vi "Open Relays.vi"(8 "error in (no error)":errorcluster, 9 "nodePath":string, 10 "NIVS.System Definition Root":refnum<k24>, 11 "WorkspaceManager in":T1) -> (0 "error out":errorcluster, 3 "WorkspaceManager out":T1)   [LabVIEW 2013]
uses:
  NationalInstruments.VeriStand.SystemStorage
  <vilib>/NI Veristand/Execution/Workspace/WorkspaceAPI.ctl
  NationalInstruments.VeriStand.ClientAPI
  NationalInstruments.VeriStand
  <vilib>/NI Veristand/Execution/Workspace/NI VeriStand - Set Single Channel Value.vi
  <vilib>/NI Veristand/Execution/Workspace/NI_VS Workspace ExecutionAPI.lvlib
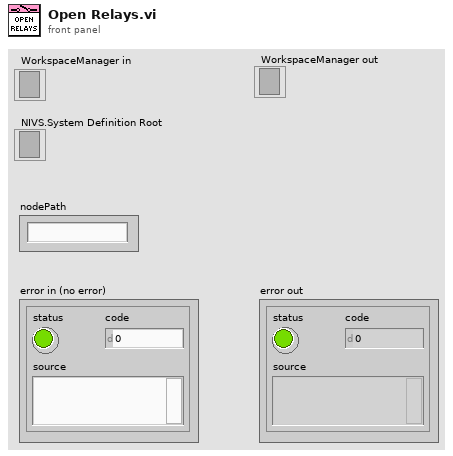
[diagram p1: front panel]
types:
  T1 = typedef "NI_VS Workspace ExecutionAPI.lvlib/WorkspaceAPI.ctl" = refnum<k24>
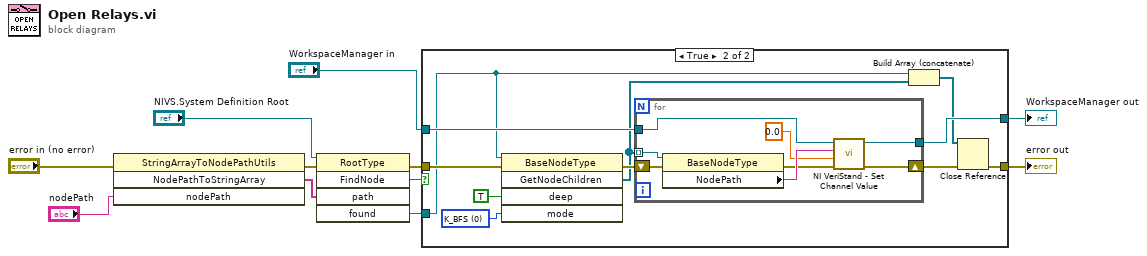
[diagram p0: block diagram]
diagram:
  n1 = invoke class="StringArrayToNodePathUtils" method="NodePathToStringArray"(error in="error in (no error)", "nodePath"="nodePath") -> (error out=w10:errorcluster, "NodePathToStringArray"=w11:string[])  [unwired: 2 in, 2 out]
  n2 = invoke class="RootType" method="FindNode"(reference="NIVS.System Definition Root", error in=w10, "path"=w11) -> (error out=w9:errorcluster, "FindNode"=w6:bool, "found"=w5:refnum<k24>)  [unwired: 2 in, 2 out]
  n3 = case shown="True" w6 {
    tunnel: w9 -> [w13 w24]
    tunnel: w5 -> [_ w16]
    tunnel: "WorkspaceManager in" -> [w12 w20]
    tunnel: [w12 w19] -> w3
    tunnel: [w13 w17] -> w2
    frame False {
    }
    frame True {
      w22 = 0 items=["K_BFS", "K_DFS", "K_CHILDONLY", "K_UP"] ("mode")
      n4 = invoke class="BaseNodeType" method="GetNodeChildren"(reference=w16, error in=w24, "deep"=TRUE, "mode"=w22) -> (error out=w21:errorcluster, "GetNodeChildren"=w15:refnum<k24>[])  [unwired: 1 in, 3 out]
      n5 = for {
        tunnel: w15 -> [w32] mode=indexing
        shift-right: [w28] -> w18
        shift-left: w21 -> [w31]
        tunnel: w20 -> [w30]
        tunnel: [w29] -> w19
        n6 = property class="BaseNodeType"(reference=w32, error in=w31) -> (error out=w26:errorcluster, "NodePath"=w27:string)  [unwired: 1 out]
        n7 = call-poly <vilib>:"NI VeriStand - Set Channel Value.vi"("error in (no error)"=w26, "Value"=0.0, "Channel"=w27, "WorkspaceManager in"=w30) -> ("error out"=w28:errorcluster, "WorkspaceManager out"=w29:T1)  [unwired: 6 in]
      }
      n8 = Build Array (concatenate)(w16, w15) -> (w14:refnum<k24>[])
      n9 = Close Reference(reference=w14, error in (no error)=w18) -> (error out=w17:errorcluster)
    }
  }
  "WorkspaceManager out" <- w3
  "error out" <- w2
